vi "2010v Calculator LabVIEW Advantage Youtube.vi"() -> ()   [LabVIEW 2010]
panel:
  in  "Calculator UI":T1
  out "Calculator Display":string
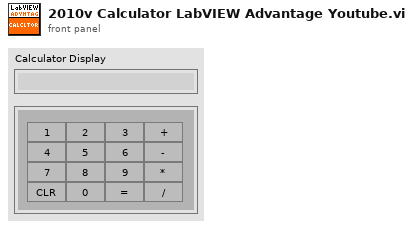
[diagram p1: front panel]
types:
  T1 = cluster{"1":bool, "2":bool, "3":bool, "Add":bool, "4":bool, "5":bool, "6":bool, "Subtract":bool, "7":bool, "8":bool, "9":bool, "Result":bool, "Clear":bool, "0":bool, "Multiply":bool, "Divide":bool}
  T2 = enum16{"No Function", "Add", "Subtract", "Multiply", "Divide"}
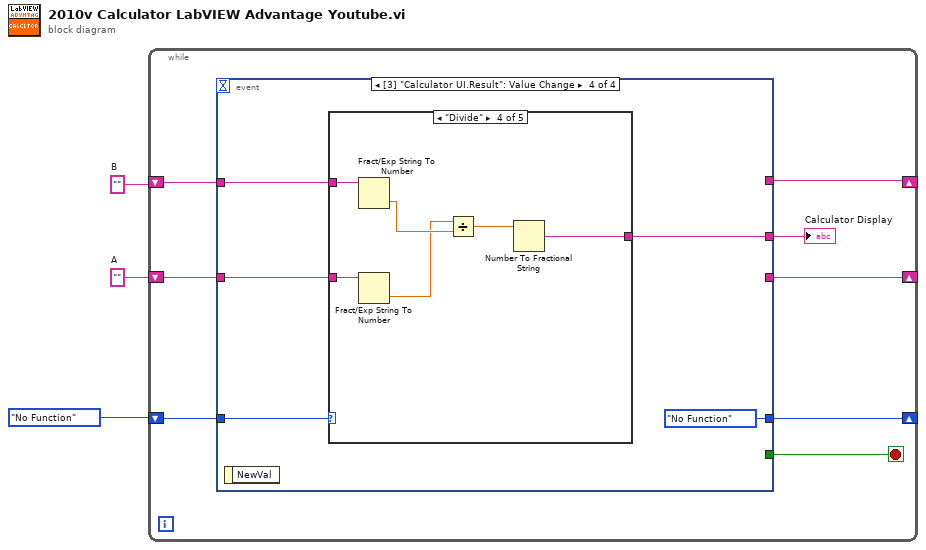
[diagram p0: block diagram]
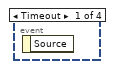
[diagram p2: hidden frame]
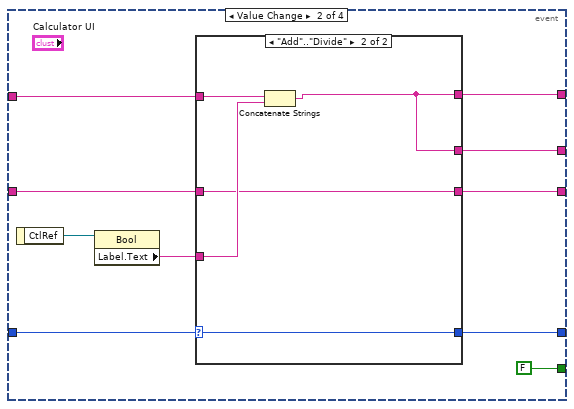
[diagram p3: hidden frame]
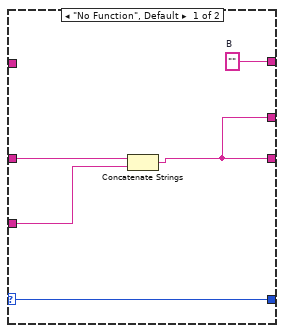
[diagram p4: hidden frame]
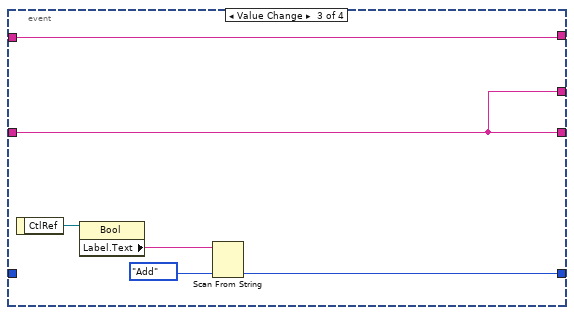
[diagram p5: hidden frame]
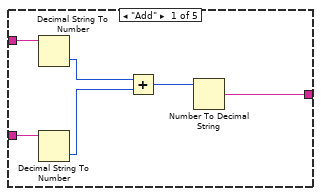
[diagram p6: hidden frame]
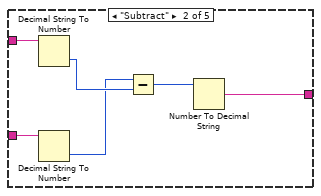
[diagram p7: hidden frame]
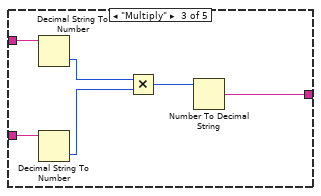
[diagram p8: hidden frame]
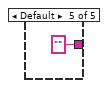
[diagram p9: hidden frame]
diagram:
  w2 = ""  # A
  w3 = ""  # B
  n1 = while {
    shift-right: [w7] -> _
    shift-left: w3 -> [w10]
    shift-right: [w6] -> _
    shift-left: w2 -> [w11]
    shift-right: [w8] -> _
    shift-left: T2."No Function" -> [w9]
    stop <- w5 stop-if-true
    n2 = event shown="[3] \"Calculator UI.Result\": Value Change" {
      selector: _ -> [_ _ _ _]
      dyn-events: _ -> [_ _ _ _]
      timeout: _ -> [_ _ _ _]
      tunnel: w11 -> [_ w19 w32 w39]
      tunnel: w10 -> [_ w13 w37 w40]
      tunnel: w9 -> [_ w20 _ w42]
      tunnel: [_ w17 w33 T2."No Function"] -> w8
      tunnel: [_ w16 w37 _] -> w7
      tunnel: [_ w15 w32 _] -> w6
      tunnel: [_ FALSE _ _] -> w5
      tunnel: [_ w12 w32 w38] -> w4
      event Timeout {
        n3 = event-data() -> ()  [unwired: 1 in, 1 out]
      }
      event "Calculator UI.1", "Calculator UI.2", "Calculator UI.3", "Calculator UI.4", "Calculator UI.5", "Calculator UI.6", "Calculator UI.7", "Calculator UI.8", "Calculator UI.9", "Calculator UI.0": Value Change {
        n4 = event-data() -> ("CtlRef"=w21:refnum<vi>)  [unwired: 1 in]
        n5 = property class="Bool"(reference=w21) -> ("Label.Text"=w18:string)  [unwired: 1 in, 2 out]
        n6 = case shown="\"Add\"..\"Divide\"" w20 {
          selector: w20 -> [w24 w28]
          tunnel: w19 -> [w26 w29]
          tunnel: w18 -> [w25 w30]
          tunnel: [w24 w28] -> w17
          tunnel: [w23 w27] -> w16
          tunnel: [w22 w29] -> w15
          tunnel: w13 -> [_ w31]
          tunnel: [w22 w27] -> w12
          frame "No Function", Default {
            w23 = ""  # B
            n7 = Concatenate Strings(w26, w25) -> (w22:string)
          }
          frame "Add".."Divide" {
            n8 = Concatenate Strings(w31, w30) -> (w27:string)
          }
        }
      }
      event "Calculator UI.Add", "Calculator UI.Subtract", "Calculator UI.Multiply", "Calculator UI.Divide": Value Change {
        n9 = event-data() -> ("CtlRef"=w36:refnum<vi>)  [unwired: 1 in]
        n10 = property class="Bool"(reference=w36) -> ("Label.Text"=w34:string)  [unwired: 1 in, 2 out]
        n11 = Scan From String "Scan From String"(input string=w34, default 1=T2."Add") -> (output 1=w33:T2)  [unwired: 3 in, 3 out]
      }
      event "Calculator UI.Result": Value Change {
        n12 = event-data() -> ()  [unwired: 1 in, 1 out]
        n13 = case shown="\"Divide\"" w42 {
          tunnel: w40 -> [w48 w54 w60 w66 _]
          tunnel: w39 -> [w47 w53 w59 w65 _]
          tunnel: [w43 w49 w55 w61 ""] -> w38
          frame "Add" {
            n14 = Decimal String To Number(string=w48) -> (number=w46:i32)  [unwired: 2 in, 1 out]
            n15 = Decimal String To Number(string=w47) -> (number=w45:i32)  [unwired: 2 in, 1 out]
            n16 = Add(x=w46, y=w45) -> (x+y=w44:i32)
            n17 = Number To Decimal String(number=w44) -> (decimal integer string=w43:string)  [unwired: 1 in]
          }
          frame "Subtract" {
            n18 = Decimal String To Number(string=w54) -> (number=w52:i32)  [unwired: 2 in, 1 out]
            n19 = Decimal String To Number(string=w53) -> (number=w51:i32)  [unwired: 2 in, 1 out]
            n20 = Subtract(x=w51, y=w52) -> (x-y=w50:i32)
            n21 = Number To Decimal String(number=w50) -> (decimal integer string=w49:string)  [unwired: 1 in]
          }
          frame "Multiply" {
            n22 = Decimal String To Number(string=w60) -> (number=w58:i32)  [unwired: 2 in, 1 out]
            n23 = Decimal String To Number(string=w59) -> (number=w57:i32)  [unwired: 2 in, 1 out]
            n24 = Multiply(x=w58, y=w57) -> (x*y=w56:i32)
            n25 = Number To Decimal String(number=w56) -> (decimal integer string=w55:string)  [unwired: 1 in]
          }
          frame "Divide" {
            n26 = Fract/Exp String To Number(string=w66) -> (number=w64:dbl)  [unwired: 3 in, 1 out]
            n27 = Fract/Exp String To Number(string=w65) -> (number=w63:dbl)  [unwired: 3 in, 1 out]
            n28 = Divide(x=w63, y=w64) -> (x/y=w62:dbl)
            n29 = Number To Fractional String(number=w62) -> (F-format string=w61:string)  [unwired: 3 in]
          }
          frame Default {
          }
        }
      }
    }
    "Calculator Display" <- w4
  }
